vi "Read From Grad PieChart.vi"(8 "error in (no error)":errorcluster caption="错误输入（无错误）", 11 "Gradient PieChart输入":refnum<class "Gradient PieChart.lvclass">) -> (0 "error out":errorcluster caption="错误输出", 2 "Grad PieChart":picture, 3 "Gradient PieChart输出":refnum<class "Gradient PieChart.lvclass">)   [LabVIEW 2012, in "Picture Box Tools.lvlib" / "Gradient PieChart.lvclass"]
uses:
  Gradient PieChart.lvclass
  Gradient PieChart.lvclass/Gradient PieChart.ctl
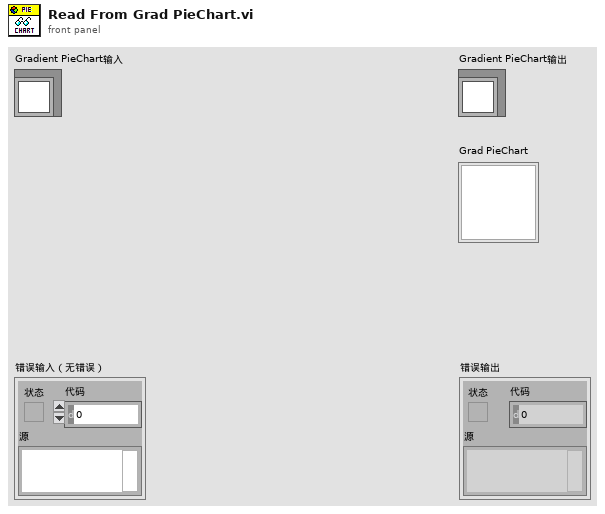
[diagram p1: front panel]
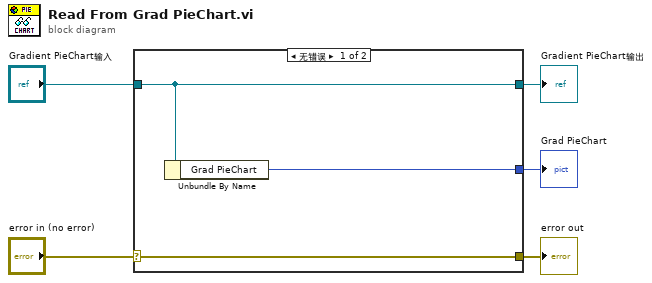
[diagram p0: block diagram]
diagram:
  n1 = case shown="无错误" "error in (no error)" {
    selector: "error in (no error)" -> [w8 w9]
    tunnel: [w8 w9] -> w4
    tunnel: [w7 w10] -> w2
    tunnel: "Gradient PieChart输入" -> [w7 w10]
    tunnel: [w6 _] -> w1
    frame No Error {
      n2 = Unbundle By Name(w7) -> ("Grad PieChart"=w6:picture)
    }
    frame Error {
    }
  }
  "error out" <- w4
  "Gradient PieChart输出" <- w2
  "Grad PieChart" <- w1
